vi "SNRStructure_ChangePowerFreq.vi"(8 "Analyze SNR Input":T1={"Pins"=["Xout"], "Published Data Id"=[], "frequency range"={"start frequency"=-1.0, "stop frequency"=-1.0}}, 9 "RFSG Input":T2={"LO configure setting"={"Carrier Frequency (Hz)"=5180000000.0, "Power Level(dBm)"=-10.0, "External Attenuation (dB)"=0.0}, "Port"=""} {"LO configure setting"."Carrier Frequency (Hz)" format="%#_6p"}, 10 "Scope Input":T3={"Min. Sample Rate"=1000000.0, "Min Record Length"=1000, "Vertical Coupling"=1, "Vertical Range (V)"=2.0, "Pins"=["Xout"]} {"Vertical Range (V)" format="%_3g"; "Vertical Coupling" items=["AC", "DC", "Ground"]; "Min. Sample Rate" format="%#_6p"}, 11 "Semiconductor Module Context":T4) -> (0 "error out":errorcluster)   [LabVIEW 2014]
uses:
  <vilib>/NI_TestStand_SemiconductorModule/NI_TestStand_Semiconductor_Module.lvlibp/PinMap/General/SemiconductorModuleContext.ctl
  Control/Scope Input.ctl
  Control/RFSG Input.ctl
  Control/Digitizier Analyze Input.ctl
  Control/Quene Type_Digitizer.ctl
  <vilib>/NI_TestStand_SemiconductorModule/NI_TestStand_Semiconductor_Module.lvlibp
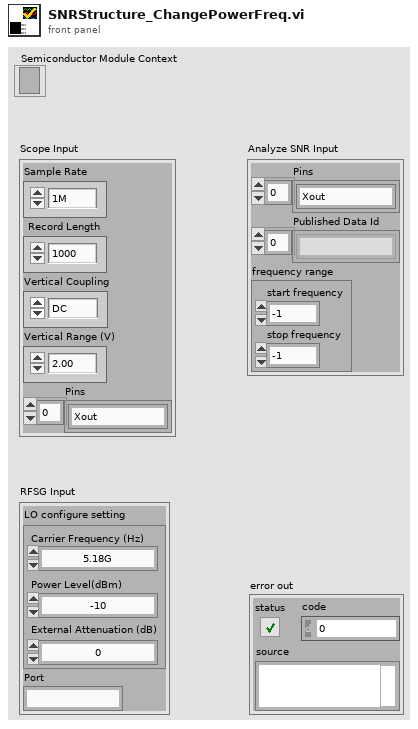
[diagram p1: front panel]
types:
  T1 = typedef "Digitizier Analyze Input.ctl" = cluster{"Pins":string[], "Published Data Id":string[], "frequency range":cluster{"start frequency":dbl, "stop frequency":dbl}}
  T2 = typedef "RFSG Input.ctl" = cluster{"LO configure setting":cluster{"Carrier Frequency (Hz)":dbl, "Power Level(dBm)":dbl, "External Attenuation (dB)":dbl}, "Port":string}
  T3 = typedef "Scope Input.ctl" = cluster{"Min. Sample Rate":dbl, "Min Record Length":i32, "Vertical Coupling":i32, "Vertical Range (V)":dbl, "Pins":string[]}
  T4 = typedef "NI_TestStand_Semiconductor_Module.lvlibp/SemiconductorModuleContext.ctl" = refnum<k7>
  T5 = typedef "Quene Type_Digitizer.ctl" = cluster{"Actiion":enum16{"Exit", "Analyze"}, "Waveform Data":waveform(dbl)[]}
  T6 = cluster{"Carrier Frequency (Hz)":dbl, "Power Level(dBm)":dbl, "External Attenuation (dB)":dbl}
  T7 = cluster{"start frequency":dbl, "stop frequency":dbl}
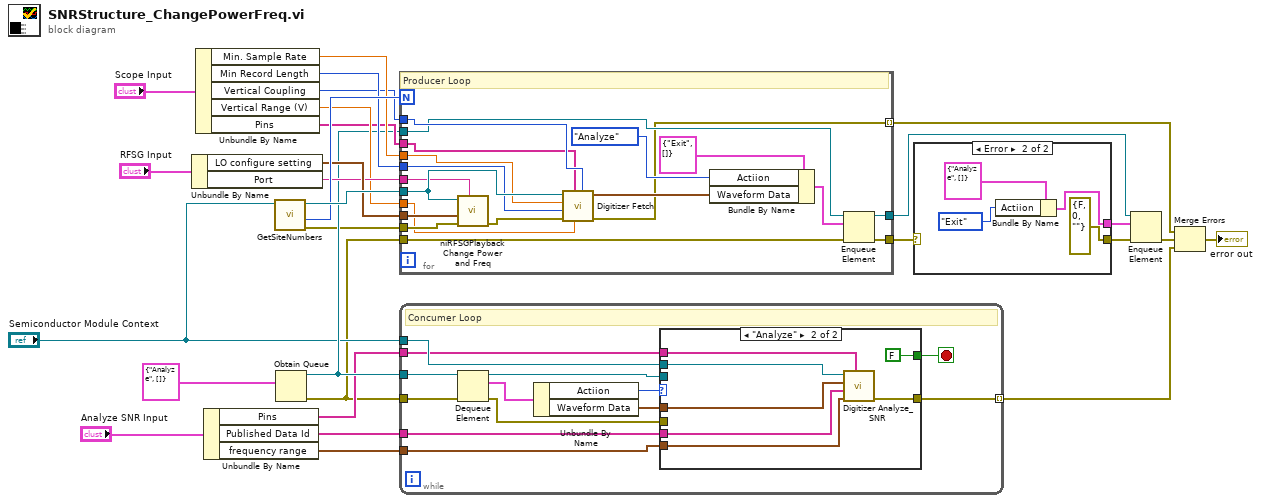
[diagram p0: block diagram]
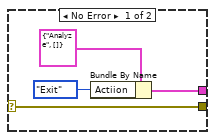
[diagram p2: hidden frame]
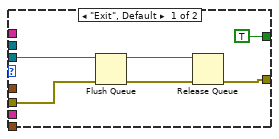
[diagram p3: hidden frame]
diagram:
  n1 = Unbundle By Name("RFSG Input") -> ("LO configure setting"=w24:T6, "Port"=w23:string)
  n2 = Unbundle By Name("Scope Input") -> ("Min. Sample Rate"=w21:dbl, "Min Record Length"=w20:i32, "Vertical Coupling"=w18:i32, "Vertical Range (V)"=w19:dbl, "Pins"=w17:string[])
  n3 = Unbundle By Name("Analyze SNR Input") -> ("Pins"=w9:string[], "Published Data Id"=w10:string[], "frequency range"=w11:T7)
  n4 = call <vilib>:"GetSiteNumbers.vi"("Semiconductor Module Context"="Semiconductor Module Context") -> ("error out"=w14:errorcluster, "Number Of Sites"=w26:i32, "Semiconductor Module Context Out"=w27:T4)  [unwired: 7 in, 1 out]
  n5 = Obtain Queue(element data type=T5 {"Actiion"=enum."Analyze", "Waveform Data"=[]}) -> (queue out=w15:refnum<queue>, error out=w4:errorcluster)  [unwired: 4 in, 1 out]
  n6 = for {
    N: w26 -> [_]
    tunnel: w27 -> [w46]
    tunnel: w24 -> [w45]
    tunnel: w23 -> [w44]
    tunnel: w21 -> [w43]
    tunnel: w20 -> [w42]
    tunnel: w19 -> [w40]
    tunnel: w18 -> [w39]
    tunnel: w17 -> [w38]
    tunnel: w15 -> [w37]
    tunnel: [w31] -> w16
    tunnel: w14 -> [w47]
    tunnel: [w29] -> w5 mode=indexing
    tunnel: w4 -> [w30]
    tunnel: [w32] -> w3
    # "Producer Loop"
    n7 = call "niRFSGPlayback Change Power and Freq.vi"("Port"=w44, "error in (no error)"=w47, "LO configure setting"=w45, "TSM Context"=w46) -> ("error out"=w41:errorcluster)  [unwired: 7 in]
    n8 = call "Digitizer Fetch.vi"("Vertical Coupling"=w39, "Vertical Range (V)"=w40, "Pins"=w38, "error in (no error)"=w41, "Min Record Length"=w42, "Min. Sample Rate"=w43, "Semiconductor Module Context"=w46) -> ("error out"=w29:errorcluster, "Waveform Data Out"=w35:waveform(dbl)[])  [unwired: 3 in]
    n9 = Bundle By Name(cluster=T5 {"Actiion"=enum."Exit", "Waveform Data"=[]}, "Actiion"=enum16{"Exit", "Analyze"}."Analyze", "Waveform Data"=w35) -> (w33:T5)
    n10 = Enqueue Element(queue=w37, element=w33, error in (no error)=w30) -> (queue out=w31:refnum<queue>, error out=w32:errorcluster)  [unwired: 1 in, 1 out]
  }
  n11 = while {
    tunnel: w15 -> [w60]
    tunnel: "Semiconductor Module Context" -> [w55]
    tunnel: w11 -> [w53]
    tunnel: w10 -> [w52]
    tunnel: w9 -> [w51]
    tunnel: w4 -> [w59]
    tunnel: [w48] -> w6 mode=indexing
    stop <- w56 stop-if-true
    # "Concumer Loop"
    n12 = Dequeue Element(queue=w60, error in (no error)=w59) -> (queue out=w50:refnum<queue>, element=w58:T5, error out=w49:errorcluster)  [unwired: 1 in, 1 out]
    n13 = Unbundle By Name(w58) -> ("Actiion"=w57:enum16{"Exit", "Analyze"}, "Waveform Data"=w54:waveform(dbl)[])
    n14 = case shown="\"Analyze\"" w57 {
      tunnel: [TRUE FALSE] -> w56
      tunnel: w55 -> [_ w72]
      tunnel: w54 -> [_ w71]
      tunnel: w53 -> [_ w70]
      tunnel: w52 -> [_ w69]
      tunnel: w51 -> [_ w68]
      tunnel: w50 -> [w63 _]
      tunnel: w49 -> [w62 _]
      tunnel: [w61 w67] -> w48
      frame "Exit", Default {
        n15 = Flush Queue(queue=w63, error in (no error)=w62) -> (queue out=w65:refnum<queue>, error out=w64:errorcluster)  [unwired: 1 out]
        n16 = Release Queue(queue=w65, error in (no error)=w64) -> (error out=w61:errorcluster)  [unwired: 1 in, 2 out]
      }
      frame "Analyze" {
        n17 = call "Digitizer Analyze_SNR.vi"("Pins"=w68, "frequency range"=w70, "Published Data Id"=w69, "Waveform Data In"=w71, "Semiconductor Module Context"=w72) -> ("error out"=w67:errorcluster)  [unwired: 3 in, 3 out]
      }
    }
  }
  n18 = case shown="Error" w3 {
    selector: w3 -> [w74 _]
    tunnel: [w75 w78] -> w2
    tunnel: [w74 errorcluster {"status"=FALSE, "code"=0, "source"=""} ("error IO")] -> w1
    frame No Error {
      n19 = Bundle By Name(cluster=T5 {"Actiion"=enum."Analyze", "Waveform Data"=[]}, "Actiion"=enum16{"Exit", "Analyze"}."Exit") -> (w75:T5)
    }
    frame Error {
      n20 = Bundle By Name(cluster=T5 {"Actiion"=enum."Analyze", "Waveform Data"=[]}, "Actiion"=enum16{"Exit", "Analyze"}."Exit") -> (w78:T5)
    }
  }
  n21 = Enqueue Element(queue=w16, element=w2, error in (no error)=w1) -> (error out=w7:errorcluster)  [unwired: 1 in, 2 out]
  n22 = Merge Errors(w5, w7, w6) -> (→"error out":errorcluster)
